vi "Remove Header.vi"(8 "error in (no error)":errorcluster, 10 "header":string(combo)="User-Agent", 11 "HTTP Client Abstract in":refnum<class "HTTP Client reqwest.lvclass">) -> (0 "error out":errorcluster, 3 "HTTP Client Abstract out":refnum<class "HTTP Client reqwest.lvclass">)   [LabVIEW 2020, in "HTTP Client reqwest.lvclass"]
uses:
  HTTP Client reqwest.lvclass
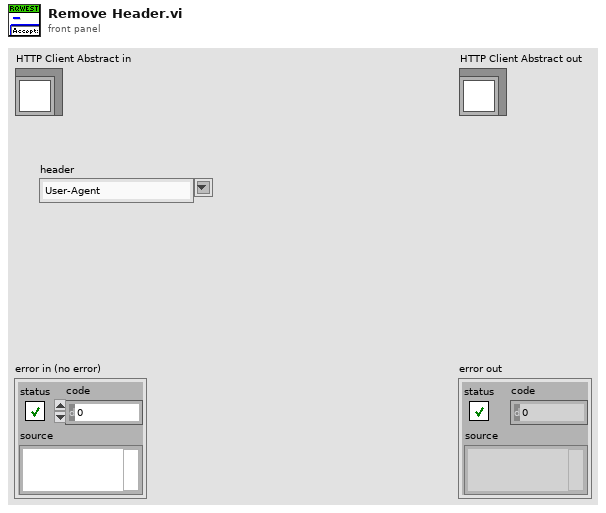
[diagram p1: front panel]
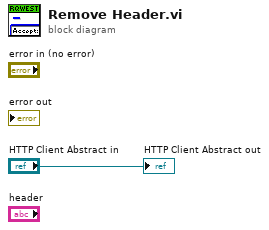
[diagram p0: block diagram]
diagram:
  "HTTP Client Abstract out" <- "HTTP Client Abstract in"
